vi "test_connection.vi"(0 "Username":string, 1 "Password":string) -> (6 "Connection Successful":bool)   [LabVIEW 2019]
uses:
  ParametersGlobal.vi
panel:
  out "standard error":string
  out "standard output":string
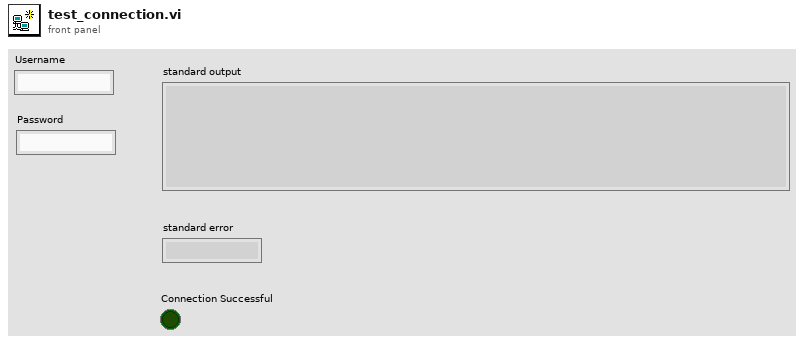
[diagram p1: front panel]
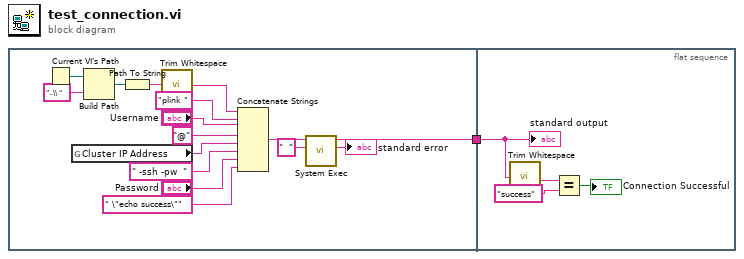
[diagram p0: block diagram]
diagram:
  n1 = flat-sequence {
    tunnel: [w6] -> w1
    tunnel: w1 -> [w20]
    frame #0 {
      n2 = Current VI's Path() -> (path=w13:path)
      n3 = global read "ParametersGlobal.vi" "Cluster IP Address"() -> (w2:string)
      n4 = Build Path(base path=w13, name or relative path="..\\ ") -> (appended path=w15:path)
      n5 = Path To String(path=w15) -> (string=w16:string)
      n6 = call <vilib>:"Trim Whitespace.vi"("string"=w16) -> ("trimmed string"=w17:string)  [unwired: 1 in]
      n7 = Concatenate Strings(w17, "plink ", "Username", "@", w2, " -ssh -pw  ", "Password", " \"echo success\"") -> (w10:string)
      n8 = call <vilib>:"System Exec.vi"("standard input"="  ", "command line"=w10) -> ("standard error"=→"standard error":string, "standard output"=w6:string)  [unwired: 6 in, 2 out]
    }
    frame #1 {
      n9 = call <vilib>:"Trim Whitespace.vi"("string"=w20) -> ("trimmed string"=w21:string)  [unwired: 1 in]
      n10 = Equal?(x=w21, y="success") -> (x = y?=→"Connection Successful":bool)
      "standard output" <- w20
    }
  }
